vi "Actor Core.vi"(8 "error in":errorcluster, 11 "Analyze Actor in":refnum<class "Analyze Actor.lvclass">) -> (0 "error out":errorcluster, 3 "Actor out":refnum<class "Actor.lvclass">)   [LabVIEW 2020, in "Analyze Actor.lvlib" / "Analyze Actor.lvclass"]
doc: "(<B>Filename</B>: Actor Framework.lvlib:Actor.lvclass:Actor Core.vi)\n\nReceives messages to the actor, reacts to them, and initiates any error handling that may shut the actor down.\n\nDescendant classes may override this VI to append parallel tasks for the actor to complete while it handles messages. Overrides use the Call Parent Method node."
uses:
  Analyze Actor.lvclass
  C:/Program Files (x86)/National Instruments/LabVIEW 2020/vi.lib/ActorFramework/Actor/Actor.lvclass
  <vilib>/ActorFramework/Actor/Actor.lvclass
  Display Actors/HIJ Vision Display/HIJ Vision Display/Analyze.ctl
  <vilib>/vision/Image Controls.llb/IMAQ Image.ctl
  Analyze Classes/Analyze BaseClass/Analyze BaseClass/Analyze BaseClass.lvclass
  Results and Overlays/Results Base/Analyze Results Base.lvclass
  <vilib>/ActorFramework/Actor/Actor.lvclass/Actor.ctl
  Analyze Actor.lvclass/Analyze Actor.ctl
  <vilib>/ActorFramework/Message Enqueuer/Message Enqueuer.lvclass/Message Enqueuer.ctl
  <vilib>/ActorFramework/Report Error Msg/Report Error Msg.lvclass/Report Error Msg.ctl
  <vilib>/ActorFramework/Message Enqueuer/Init from Existing Queue.vi
  <vilib>/ActorFramework/Message Enqueuer/Enqueue.vi
  <vilib>/ActorFramework/Report Error Msg/Report Error Msg.lvclass
  C:/Program Files (x86)/National Instruments/LabVIEW 2020/vi.lib/ActorFramework/Message/Message.lvclass
  <vilib>/ActorFramework/Message Priority Queue/Priority Enqueue.vi
  <vilib>/ActorFramework/Message Enqueuer/Message Enqueuer.lvclass
panel:
  in  "StopSignal":bool=TRUE
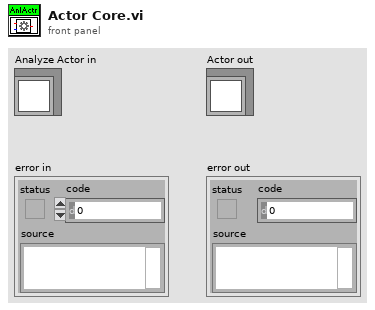
[diagram p1: front panel]
types:
  T1 = typedef "Analyze Actor.lvlib/Analyze Actor.lvclass/Analyze.ctl" = cluster{"Image":T2, "ImageNr":i32, "Analyze Objects":refnum<class "Analyze BaseClass.lvclass">[], "Pre Results":refnum<class "Analyze Results Base.lvclass">[]}
  T2 = typedef "IMAQ Image.ctl" = refnum<image>
  T3 = typedef "Image Type" = u32
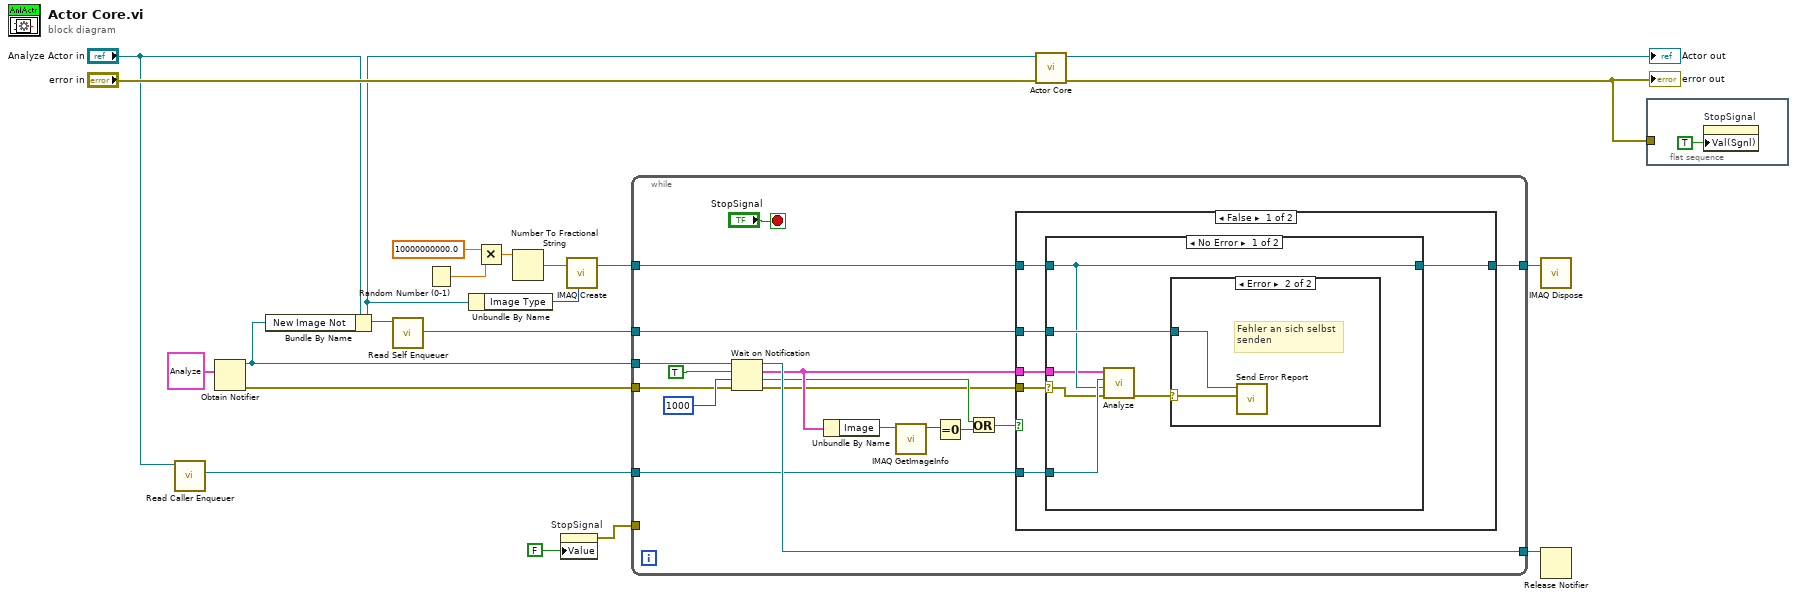
[diagram p0: block diagram]
diagram:
  n1 = call <vilib>:"Read Caller Enqueuer.vi"("Actor"="Analyze Actor in") -> ("Caller Enqueuer"=w2:refnum<class "Message Enqueuer.lvclass">)  [unwired: 10 in]
  n2 = Obtain Notifier(notification data type=T1 {"Image"=refnum, "ImageNr"=0, "Analyze Objects"=[], "Pre Results"=[]}) -> (notifier out=w11:refnum<notifier>, error out=w15:errorcluster)  [unwired: 3 in, 1 out]
  n3 = Bundle By Name(cluster="Analyze Actor in", "New Image Not"=w11) -> (w1:refnum<class "Analyze Actor.lvclass">)
  n4 = call <vilib>:"Read Self Enqueuer.vi"("Actor"=w1) -> ("Self Enqueuer"=w4:refnum<class "Message Enqueuer.lvclass">)  [unwired: 10 in]
  n5 = Random Number (0-1)() -> (number: 0 to 1=w10:dbl)
  n6 = Unbundle By Name(w1) -> ("Image Type"=w17:T3)
  n7 = Multiply(x=10000000000.0, y=w10) -> (x*y=w9:dbl)
  n8 = Number To Fractional String(number=w9) -> (F-format string=w8:string)  [unwired: 3 in]
  n9 = property on="StopSignal" class="Bool (strict)"("Value"=FALSE ("Value (Signaling)")) -> (error out=w16:errorcluster)  [unwired: 2 in, 1 out]
  n10 = call "IMAQ Create"("Image Name"=w8, "Image Type"=w17) -> ("New Image"=w7:T2)  [unwired: 3 in, 1 out]
  n11 = while {
    tunnel: w11 -> [w32]
    tunnel: w15 -> [w36]
    tunnel: w16 -> [_]
    tunnel: w4 -> [w34]
    tunnel: [w31] -> w13
    tunnel: w2 -> [w30]
    tunnel: w7 -> [w29]
    tunnel: [w28] -> w6
    stop <- "StopSignal" stop-if-true
    n12 = Wait on Notification(notifier=w32, ignore previous (F)=TRUE, timeout in ms (-1)=1000, error in (no error)=w36) -> (notifier out=w31:refnum<notifier>, notification=w27:T1, timed out?=w22:bool, error out=w21:errorcluster)
    n13 = Unbundle By Name(w27) -> ("Image"=w26:T2)
    n14 = call "IMAQ GetImageInfo"("Image"=w26) -> ("X Resolution"=w25:i32)  [unwired: 3 in, 7 out]
    n15 = Equal To 0?(x=w25) -> (x = 0?=w23:bool)
    n16 = Or(x=w22, y=w23) -> (x .or. y?=w24:bool)
    n17 = case shown="False" w24 {
      tunnel: w27 -> [w42 _]
      tunnel: w34 -> [w41 _]
      tunnel: w21 -> [w43 _]
      tunnel: w30 -> [w40 _]
      tunnel: w29 -> [w39 w53]
      tunnel: [w38 w53] -> w28
      frame False {
        n18 = case shown="No Error" w43 {
          selector: w43 -> [w48 _]
          tunnel: w42 -> [w44 _]
          tunnel: w41 -> [w46 _]
          tunnel: w40 -> [w49 _]
          tunnel: w39 -> [w45 w52]
          tunnel: [w45 w52] -> w38
          frame No Error {
            n19 = call "Analyze.vi"("error in (no error)"=w48, "Work Image"=w45, "Destination"=w49, "Analyze Data"=w44) -> ("error out"=w47:errorcluster)  [unwired: 7 in]
            n20 = case shown="Error" w47 {
              selector: w47 -> [_ w51]
              tunnel: w46 -> [_ w50]
              frame No Error {
              }
              frame Error {
                # "Fehler an sich selbst\nsenden"
                n21 = call <vilib>:"Send Error Report.vi"("Error From Sender"=w51, "Message Enqueuer"=w50) -> ()  [unwired: 9 in, 1 out]
              }
            }
          }
          frame Error {
          }
        }
      }
      frame True {
      }
    }
  }
  n22 = call-parent "Actor Core.vi"("error in"="error in", "Actor in"=w1) -> ("error out"=w18:errorcluster, "Actor out"=→"Actor out":refnum<class "Actor.lvclass">)  [unwired: 8 in]
  "error out" <- w18
  n23 = call "IMAQ Dispose"("Image"=w6) -> ()  [unwired: 5 in, 1 out]
  n24 = Release Notifier(notifier=w13) -> ()  [unwired: 2 in, 3 out]
  n25 = flat-sequence {
    tunnel: w18 -> [_]
    frame #0 {
      n26 = property on="StopSignal" class="Bool (strict)"("Val(Sgnl)"=TRUE ("Value (Signaling)")) -> ()  [unwired: 2 in, 2 out]
    }
  }
